vi "CMNDI.vi"(10 "K":T2) -> (0 "ClearAcc":bool, 1 "Exec":bool, 2 "Func":T1, 3 "SelOp":bool, 4 "Cread":bool, 5 "Wr":bool, 6 "Read":bool, 7 "SelInp":bool)   [LabVIEW 2017]
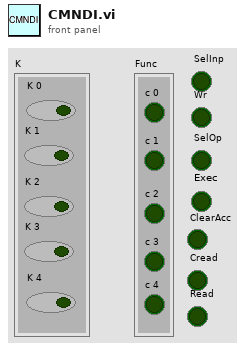
[diagram p1: front panel]
types:
  T1 = cluster{"c 0":bool, "c 1":bool, "c 2":bool, "c 3":bool, "c 4":bool}
  T2 = cluster{"K 0":bool, "K 1":bool, "K 2":bool, "K 3":bool, "K 4":bool}
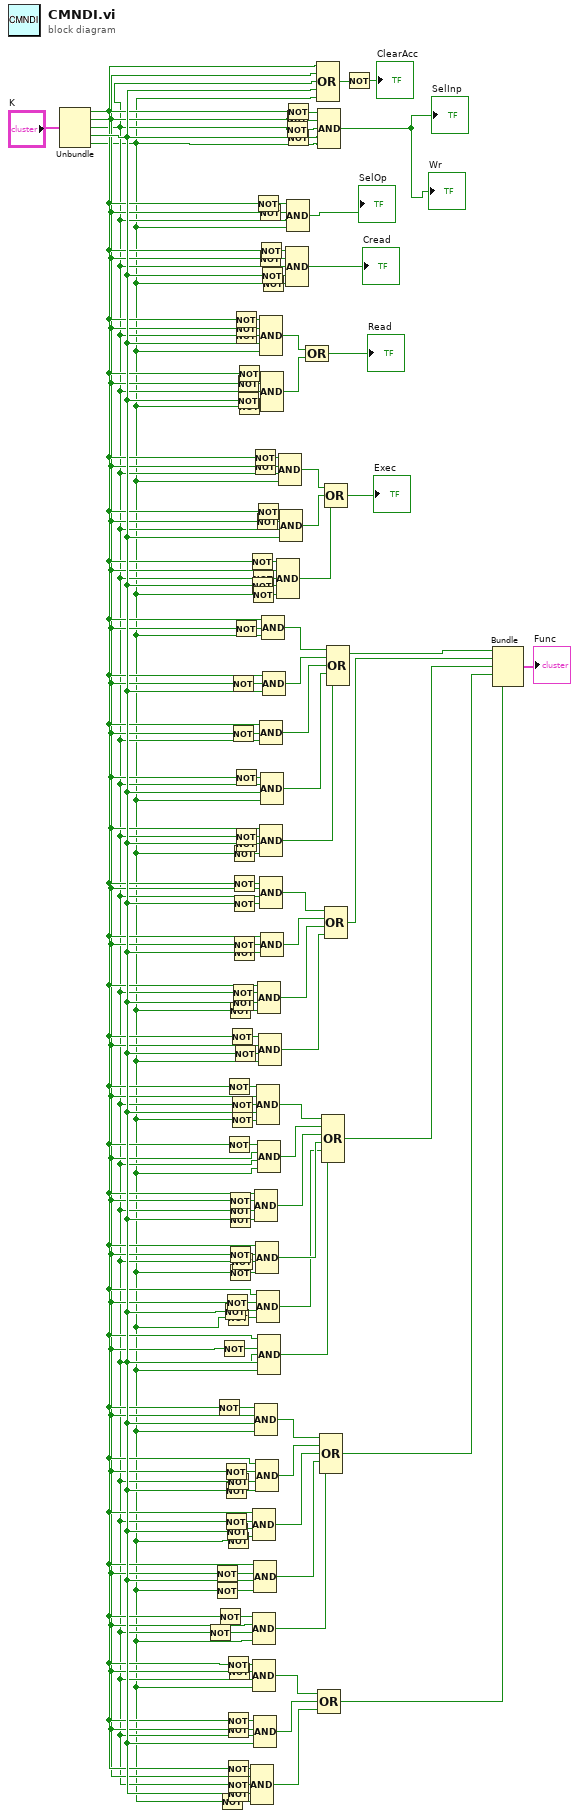
[diagram p0: block diagram]
diagram:
  n1 = Unbundle("K") -> ("K 0"=w5:bool, "K 1"=w4:bool, "K 2"=w3:bool, "K 3"=w8:bool, "K 4"=w2:bool)
  n2 = Not(x=w3) -> (.not. x?=w6:bool)
  n3 = Not(x=w4) -> (.not. x?=w10:bool)
  n4 = Not(x=w2) -> (.not. x?=w9:bool)
  n5 = Not(x=w5) -> (.not. x?=w15:bool)
  n6 = Not(x=w5) -> (.not. x?=w7:bool)
  n7 = Not(x=w2) -> (.not. x?=w44:bool)
  n8 = Not(x=w4) -> (.not. x?=w24:bool)
  n9 = Not(x=w8) -> (.not. x?=w26:bool)
  n10 = Not(x=w4) -> (.not. x?=w17:bool)
  n11 = Not(x=w8) -> (.not. x?=w14:bool)
  n12 = Not(x=w3) -> (.not. x?=w16:bool)
  n13 = Not(x=w4) -> (.not. x?=w25:bool)
  n14 = Not(x=w8) -> (.not. x?=w12:bool)
  n15 = Not(x=w2) -> (.not. x?=w27:bool)
  n16 = Not(x=w3) -> (.not. x?=w13:bool)
  n17 = Not(x=w2) -> (.not. x?=w11:bool)
  n18 = Not(x=w5) -> (.not. x?=w53:bool)
  n19 = Not(x=w5) -> (.not. x?=w49:bool)
  n20 = Not(x=w4) -> (.not. x?=w48:bool)
  n21 = Not(x=w5) -> (.not. x?=w47:bool)
  n22 = Not(x=w3) -> (.not. x?=w46:bool)
  n23 = Not(x=w8) -> (.not. x?=w45:bool)
  n24 = Not(x=w5) -> (.not. x?=w40:bool)
  n25 = Not(x=w5) -> (.not. x?=w32:bool)
  n26 = Not(x=w4) -> (.not. x?=w50:bool)
  n27 = Not(x=w2) -> (.not. x?=w59:bool)
  n28 = Not(x=w4) -> (.not. x?=w39:bool)
  n29 = Not(x=w3) -> (.not. x?=w38:bool)
  n30 = Not(x=w8) -> (.not. x?=w31:bool)
  n31 = Not(x=w4) -> (.not. x?=w29:bool)
  n32 = Not(x=w2) -> (.not. x?=w28:bool)
  n33 = Not(x=w5) -> (.not. x?=w58:bool)
  n34 = Not(x=w3) -> (.not. x?=w34:bool)
  n35 = Not(x=w2) -> (.not. x?=w33:bool)
  n36 = Not(x=w3) -> (.not. x?=w30:bool)
  n37 = Not(x=w4) -> (.not. x?=w75:bool)
  n38 = Not(x=w4) -> (.not. x?=w74:bool)
  n39 = Not(x=w3) -> (.not. x?=w61:bool)
  n40 = Not(x=w8) -> (.not. x?=w60:bool)
  n41 = Not(x=w2) -> (.not. x?=w70:bool)
  n42 = Not(x=w5) -> (.not. x?=w65:bool)
  n43 = Not(x=w8) -> (.not. x?=w64:bool)
  n44 = Not(x=w4) -> (.not. x?=w63:bool)
  n45 = Not(x=w8) -> (.not. x?=w62:bool)
  n46 = Not(x=w8) -> (.not. x?=w57:bool)
  n47 = Not(x=w5) -> (.not. x?=w90:bool)
  n48 = Not(x=w4) -> (.not. x?=w89:bool)
  n49 = Not(x=w3) -> (.not. x?=w85:bool)
  n50 = Not(x=w4) -> (.not. x?=w76:bool)
  n51 = Not(x=w4) -> (.not. x?=w73:bool)
  n52 = Not(x=w3) -> (.not. x?=w72:bool)
  n53 = Not(x=w8) -> (.not. x?=w71:bool)
  n54 = Not(x=w4) -> (.not. x?=w87:bool)
  n55 = Not(x=w8) -> (.not. x?=w84:bool)
  n56 = Not(x=w5) -> (.not. x?=w88:bool)
  n57 = Not(x=w2) -> (.not. x?=w83:bool)
  n58 = Not(x=w5) -> (.not. x?=w102:bool)
  n59 = Not(x=w8) -> (.not. x?=w100:bool)
  n60 = Not(x=w3) -> (.not. x?=w99:bool)
  n61 = Not(x=w2) -> (.not. x?=w101:bool)
  n62 = Not(x=w5) -> (.not. x?=w106:bool)
  n63 = Not(x=w4) -> (.not. x?=w105:bool)
  n64 = Compound Arithmetic op=AND(w47, w4, w46, w45, w44) -> (w54:bool)
  n65 = Not(x=w4) -> (.not. x?=w103:bool)
  n66 = Not(x=w5) -> (.not. x?=w111:bool)
  n67 = Not(x=w5) -> (.not. x?=w104:bool)
  n68 = Compound Arithmetic op=AND(w5, w16, w12, w11) -> (w20:bool)
  n69 = Compound Arithmetic op=AND(w7, w4, w6, w2) -> (w18:bool)
  n70 = Compound Arithmetic op=AND(w53, w50, w3, w2) -> (w52:bool)
  n71 = Compound Arithmetic op=AND(w5, w10, w8, w9) -> (w19:bool)
  n72 = Compound Arithmetic op=AND(w49, w48, w3, w8) -> (w55:bool)
  n73 = Not(x=w4) -> (.not. x?=w112:bool)
  n74 = Not(x=w4) -> (.not. x?=w95:bool)
  n75 = Compound Arithmetic op=AND(w5, w39, w38, w31) -> (w42:bool)
  n76 = Compound Arithmetic op=AND(w15, w4, w8, w2) -> (w22:bool)
  n77 = Not(x=w5) -> (.not. x?=w96:bool)
  n78 = Compound Arithmetic op=AND(w5, w29, w30, w28) -> (w41:bool)
  n79 = Compound Arithmetic op=AND(w5, w17, w13, w14) -> (w21:bool)
  n80 = Not(x=w8) -> (.not. x?=w93:bool)
  n81 = Compound Arithmetic op=AND(w40, w4, w34, w8, w33) -> (w37:bool)
  n82 = Compound Arithmetic op=AND(w5, w25, w26, w27) -> (w36:bool)
  n83 = Not(x=w2) -> (.not. x?=w94:bool)
  n84 = Compound Arithmetic op=AND(w5, w61, w60, w59) -> (w68:bool)
  n85 = Compound Arithmetic op=AND(w32, w4, w3, w2) -> (w43:bool)
  n86 = Compound Arithmetic op=AND(w5, w24, w3, w8, w2) -> (w35:bool)
  n87 = Compound Arithmetic op=AND(w58, w4, w57, w2) -> (w67:bool)
  n88 = Compound Arithmetic op=AND(w90, w89, w85, w8, w2) -> (w92:bool)
  n89 = Compound Arithmetic op=AND(w5, w74, w3) -> (w79:bool)
  n90 = Compound Arithmetic op=AND(w4, w72, w71, w70) -> (w77:bool)
  n91 = Compound Arithmetic op=AND(w65, w4, w3, w64) -> (w56:bool)
  n92 = Compound Arithmetic op=AND(w88, w87, w3, w84, w83) -> (w91:bool)
  n93 = Compound Arithmetic op=AND(w73, w3, w8, w2) -> (w78:bool)
  n94 = Compound Arithmetic op=AND(w5, w63, w62) -> (w69:bool)
  n95 = Compound Arithmetic op=AND(w5, w76, w2) -> (w82:bool)
  n96 = Compound Arithmetic op=AND(w5, w75, w8) -> (w81:bool)
  n97 = Compound Arithmetic op=AND(w102, w4, w99, w100, w101) -> (w107:bool)
  n98 = Compound Arithmetic op=AND(w106, w105, w3, w2) -> (w109:bool)
  n99 = Compound Arithmetic op=AND(w104, w103, w3, w8) -> (w108:bool)
  n100 = Not(x=w4) -> (.not. x?=w116:bool)
  n101 = Not(x=w3) -> (.not. x?=w115:bool)
  n102 = Not(x=w5) -> (.not. x?=w117:bool)
  n103 = Not(x=w8) -> (.not. x?=w114:bool)
  n104 = Compound Arithmetic op=AND(w96, w95, w3, w93, w94) -> (→"Cread":bool)
  n105 = Compound Arithmetic op=AND(w111, w112, w3, w2) -> (→"SelOp":bool)
  n106 = Compound Arithmetic op=OR(w92, w91) -> (→"Read":bool)
  n107 = Compound Arithmetic op=OR(w5, w4, w3, w8, w2) -> (w119:bool)
  n108 = Compound Arithmetic op=AND(w117, w116, w115, w114, w2) -> (→"SelInp" →"Wr":bool)
  n109 = Compound Arithmetic op=OR(w52, w55, w54) -> (w51:bool)
  n110 = Compound Arithmetic op=OR(w22, w21, w20, w19, w18) -> (w1:bool)
  n111 = Compound Arithmetic op=OR(w37, w43, w42, w41, w36, w35) -> (w23:bool)
  n112 = Compound Arithmetic op=OR(w109, w108, w107) -> (→"Exec":bool)
  n113 = Compound Arithmetic op=OR(w56, w69, w68, w67) -> (w66:bool)
  n114 = Compound Arithmetic op=OR(w82, w81, w79, w78, w77) -> (w80:bool)
  n115 = Not(x=w119) -> (.not. x?=→"ClearAcc":bool)
  n116 = Bundle(w80, w66, w23, w1, w51) -> (→"Func":cluster{bool, bool, bool, bool, bool})  [unwired: 1 in]
